vi "PR Switch To Thru Mode.vi"   [LabVIEW 2022 SP3, in "BS6006PRPLUS.lvlib"]
doc: "The function sets the mode of Pulser/Receiver is THRU mode for pitch-catch testing.\n\nextern \"C\" BS6006PRPLUS_API void __cdecl PR_SwitchToThruMode();"
uses:
  BS6006PRPLUS.lvlib
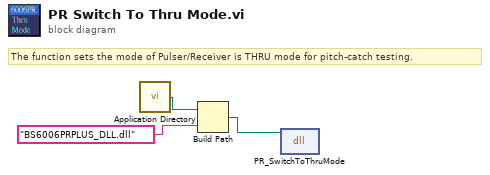
[diagram p0: block diagram]
diagram:
  # "The function sets the mode of Pulser/Receiver is THRU mode for pitch-catch testing."
  n1 = call <vilib>:"Application Directory.vi"() -> ("Application Directory"=w3:path)
  n2 = Build Path(base path=w3, name or relative path="BS6006PRPLUS_DLL.dll") -> (appended path=w1:path)
  n3 = dll-call lib="E:/Broadsound_Program/PulserReceiver/6006PR PLUS/API/DLL/LabVIEW 15/VIs/BS6006PRPLUS_DLL.dlls" fn="PR_SwitchToThruMode"(path in=w1) -> ()  [unwired: 3 in, 2 out]
